vi "zmq_rep LabVIEW server.vi"() -> ()   [LabVIEW 2019]
uses:
  <vilib>/addons/zeromq/socket_type.ctl
  erx-demo/eRX 802.15.4/Performance measure context.ctl
  <vilib>/addons/zeromq/zmq_context.lvclass
  <vilib>/addons/zeromq/zmq_socket.lvclass
  <vilib>/addons/zeromq/zeromq.lvlib
panel:
  out "data":string
  out "Measures out":T1 {"Total samples" format="%#_6p"; "Elapsed time" format="%#_6p"; "Samples per second" format="%#_6p"; "Time per sample" format="%#_6p"; "Packets per second" format="%#_6p"; "Last samples per second" format="%#_6p"}
  out "error out":errorcluster
  in  "Stop 2":bool
  in  "Stop":bool
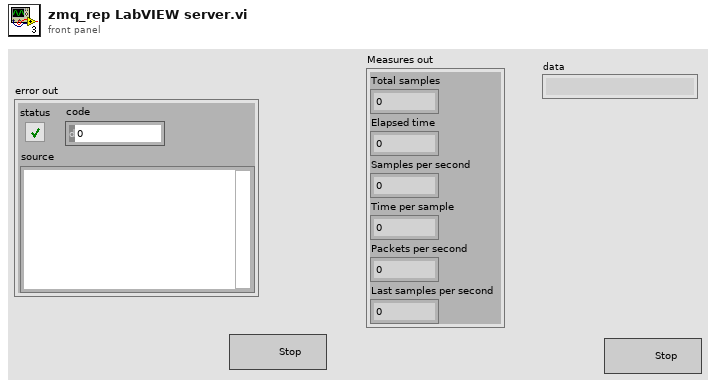
[diagram p1: front panel]
types:
  T1 = cluster{"Total samples":dbl, "Elapsed time":dbl, "Samples per second":dbl, "Time per sample":dbl, "Packets per second":dbl, "Last samples per second":dbl}
  T2 = typedef "zeromq.lvlib/socket_type.ctl" = enum8{"ZMQ_PAIR", "ZMQ_PUB", "ZMQ_SUB", "ZMQ_REQ", "ZMQ_REP", "ZMQ_DEALER", "ZMQ_ROUTER", "ZMQ_PULL", "ZMQ_PUSH", "ZMQ_XPUB", "ZMQ_XSUB"}
  T3 = typedef "Performance measure context.ctl" = cluster{"Seconds decayed":dbl, "Samples decayed":dbl, "Packet count":dbl, "Samples count":dbl, "Timestamp":dbl, "Start time":dbl}
  T4 = enum16{"Standard", "Buffered", "CRLF", "Immediate"}
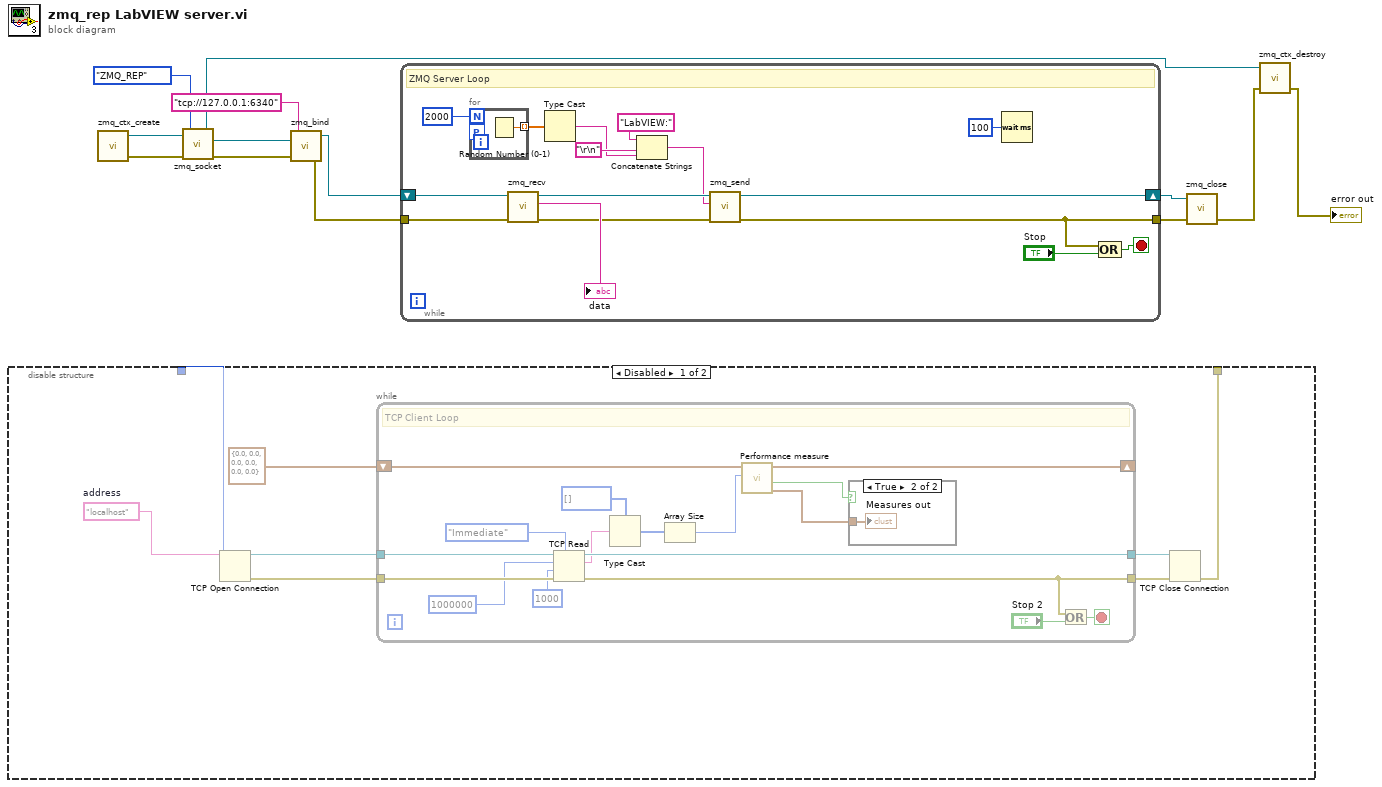
[diagram p0: block diagram]
diagram:
  n1 = disable-structure shown="Disabled" {
    disable-tunnel: [w18 _] -> _
    disable-tunnel: _ -> [w17 _]
    frame Disabled {
      w19 = "localhost"  # address
      n2 = TCP Open Connection(address=w19, remote port or service name=w17) -> (connection ID=w21:refnum<k5>, error out=w20:errorcluster)  [unwired: 3 in]
      n3 = while {
        tunnel: w20 -> [w37]
        tunnel: w21 -> [w38]
        tunnel: [w32] -> w16
        tunnel: [w31] -> w15
        shift-right: [w25] -> _
        shift-left: T3 {"Seconds decayed"=0.0, "Samples decayed"=0.0, "Packet count"=0.0, "Samples count"=0.0, "Timestamp"=0.0, "Start time"=0.0} ("Context out") -> [w24]
        stop <- w35 stop-if-true
        # "TCP Client Loop"
        n4 = TCP Read(connection ID=w38, bytes to read=1000000, error in (no error)=w37, 7:T4."Immediate" ("mode (standard)"), 9:1000 ("timeout ms (25000)")) -> (connection ID out=w32:refnum<k5>, data out=w29:string, error out=w31:errorcluster)
        n5 = Type Cast(type=u8[] [], x=w29) -> (*(type *) &x=w27:u8[])
        n6 = Array Size(array=w27) -> (size(s)=w26:i32)
        n7 = call "Performance measure.vi"("Samples processed"=w26, "Context in"=w24) -> ("Measures out"=w23:T1, "Update"=w22:bool, "Context out"=w25:T3)  [unwired: 7 in]
        n8 = case shown="True" w22 {
          tunnel: w23 -> [_ w39]
          frame False {
          }
          frame True {
            "Measures out" <- w39
          }
        }
        n9 = Or(x=w31, y="Stop 2") -> (x .or. y?=w35:bool)
      }
      n10 = TCP Close Connection(connection ID=w16, error in (no error)=w15) -> (error out=w18:errorcluster)  [unwired: 1 in, 1 out]
    }
    frame Enabled {
    }
  }
  n11 = call <vilib>:"zmq_ctx_create.vi"() -> ("error out"=w9:errorcluster, "context out"=w8:refnum<class "zmq_context.lvclass">)  [unwired: 4 in]
  n12 = call <vilib>:"zmq_socket.vi"("error in"=w9, "socket type"=socket_type."ZMQ_REP", "context in"=w8) -> ("error out"=w10:errorcluster, "socket out"=w13:refnum<class "zmq_socket.lvclass">, "context out"=w3:refnum<class "zmq_context.lvclass">)  [unwired: 2 in]
  n13 = call <vilib>:"zmq_bind.vi"("error in"=w10, "endpoint"="tcp://127.0.0.1:6340", "socket in"=w13) -> ("error out"=w11:errorcluster, "socket out"=w12:refnum<class "zmq_socket.lvclass">)  [unwired: 1 in]
  n14 = while {
    tunnel: [w46] -> w5
    tunnel: w11 -> [w50]
    shift-right: [w41] -> w4
    shift-left: w12 -> [w51]
    stop <- w55 stop-if-true
    # "ZMQ Server Loop"
    n15 = for {
      N: 2000 ("# of Points") -> [_]
      tunnel: [w56] -> w52 mode=indexing
      workers-P: _ -> [_]
      n16 = Random Number (0-1)() -> (number: 0 to 1=w56:dbl)
    }
    n17 = call <vilib>:"zmq_recv.vi"("error in"=w50, "socket in"=w51) -> ("error out"=w48:errorcluster, "data"=→"data":string, "socket out"=w47:refnum<class "zmq_socket.lvclass">)  [unwired: 3 in, 2 out]
    n18 = Type Cast(x=w52) -> (*(type *) &x=w43:string)  [unwired: 1 out]
    n19 = Concatenate Strings("LabVIEW:" ("data"), "\r\n", w43) -> (w42:string)
    n20 = call <vilib>:"zmq_send.vi"("error in"=w48, "data"=w42, "socket in"=w47) -> ("error out"=w46:errorcluster, "socket out"=w41:refnum<class "zmq_socket.lvclass">)  [unwired: 4 in]
    n21 = Wait (ms)(milliseconds to wait=u32 100) -> ()  [unwired: 1 out]
    n22 = Compound Arithmetic op=OR(w46, "Stop") -> (w55:bool)
  }
  n23 = call <vilib>:"zmq_close.vi"("error in"=w5, "socket"=w4) -> ("error out"=w2:errorcluster)  [unwired: 3 in]
  n24 = call <vilib>:"zmq_ctx_destroy.vi"("error in"=w2, "context in"=w3) -> ("error out"=→"error out":errorcluster)  [unwired: 3 in]
